vi "joysticks_to_commands.vi"(11 "Joysticks":T4) -> (3 "Commands":T1)   [LabVIEW 2012]
uses:
  <vilib>/Rock Robotics/WPI/Joystick/WPI_JoystickButtonState.ctl
  Commands.ctl
  mecanum/mecanum_control.ctl
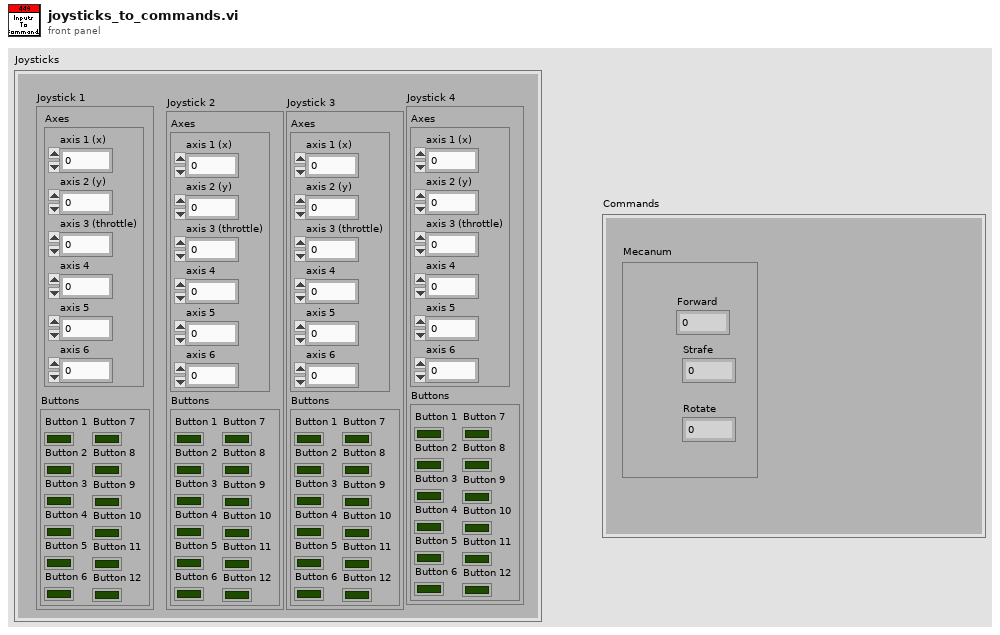
[diagram p1: front panel]
types:
  T1 = typedef "Commands.ctl" = cluster{"Mecanum":T2}
  T2 = typedef "mecanum_control.ctl" = cluster{"Forward":dbl, "Strafe":dbl, "Rotate":dbl}
  T3 = typedef "WPI_JoystickButtonState.ctl" = cluster{"Button 1":bool, "Button 2":bool, "Button 3":bool, "Button 4":bool, "Button 5":bool, "Button 6":bool, "Button 7":bool, "Button 8":bool, "Button 9":bool, "Button 10":bool, "Button 11":bool, "Button 12":bool}
  T4 = cluster{"Joystick 1":cluster{"Axes":cluster{"axis 1 (x)":dbl, "axis 2 (y)":dbl, "axis 3 (throttle)":dbl, "axis 4":dbl, "axis 5":dbl, "axis 6":dbl}, "Buttons":T3}, "Joystick 2":cluster{"Axes":cluster{"axis 1 (x)":dbl, "axis 2 (y)":dbl, "axis 3 (throttle)":dbl, "axis 4":dbl, "axis 5":dbl, "axis 6":dbl}, "Buttons":T3}, "Joystick 3":cluster{"Axes":cluster{"axis 1 (x)":dbl, "axis 2 (y)":dbl, "axis 3 (throttle)":dbl, "axis 4":dbl, "axis 5":dbl, "axis 6":dbl}, "Buttons":T3}, "Joystick 4":cluster{"Axes":cluster{"axis 1 (x)":dbl, "axis 2 (y)":dbl, "axis 3 (throttle)":dbl, "axis 4":dbl, "axis 5":dbl, "axis 6":dbl}, "Buttons":T3}}
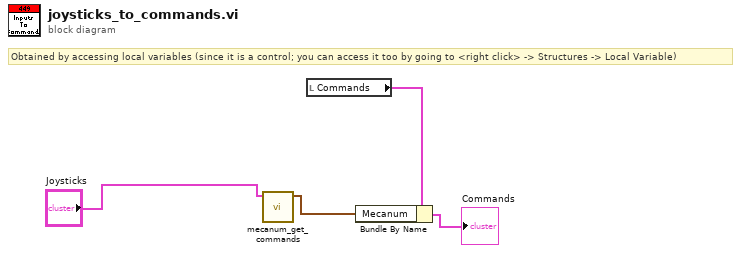
[diagram p0: block diagram]
diagram:
  # "Obtained by accessing local variables (since it is a control; you can access it too by going to <right click> -> Structures -> Local Variable)"
  n1 = call "mecanum_get_commands.vi"("Joysticks"="Joysticks") -> ("Mecanum"=w1:T2)  [unwired: 10 in]
  n2 = local read "Commands"() -> (w4:T1)
  n3 = Bundle By Name(cluster=w4, "Mecanum"=w1) -> (→"Commands":T1)
